vi "HoloLink_get_one_trajectorie.vi"(8 "error in (no error)":errorcluster, 10 "feature_number":i32, 11 "session in":refnum<k35>) -> (0 "error out":errorcluster, 2 "trajectorie":dbl[][](array[numeric]), 3 "Refnum out":refnum<k35>)   [LabVIEW 2023, in "holoPyTracks.lvlib"]
uses:
  holoPyTracks.lvlib
panel:
  # "wavelenght, optical_index, image_size_X, image_size_Y, pixel_size, magnification = holo_info\n\n    propag_param, focus_param, binarisation_param, CCL_param = analyse_parameters\n    distance_ini, nb_plane, propag_step, filter = propag_param\n    high_pass_filter, low_pass_filter = filter\n    #focus parameters unpacking\n    focus_type, sum_size = focus_param\n    #binarisation parameters unpacking\n    nbStdVarThreshold, threshold_target = binarisation_param\n    #CCL parameters unpacking\n    n_connectivity, min_voxel, max_voxel = CCL_param"
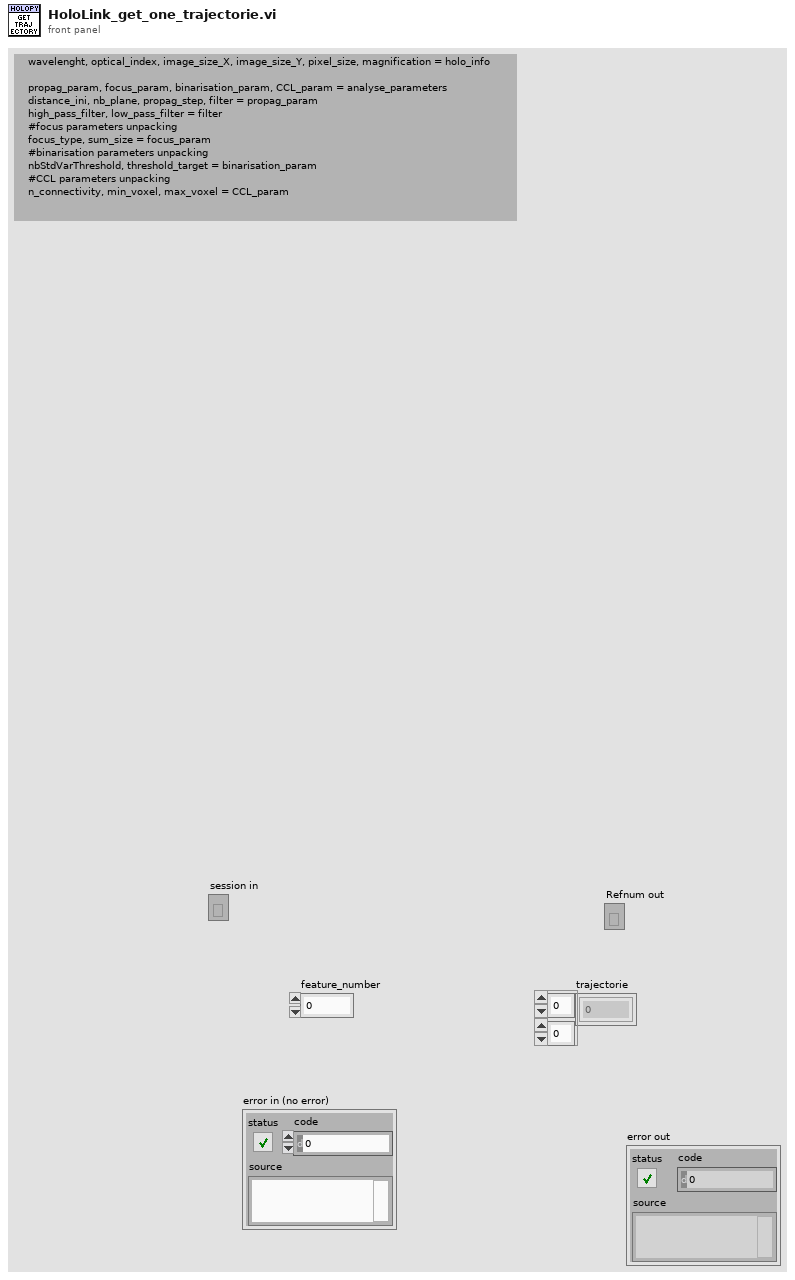
[diagram p1: front panel]
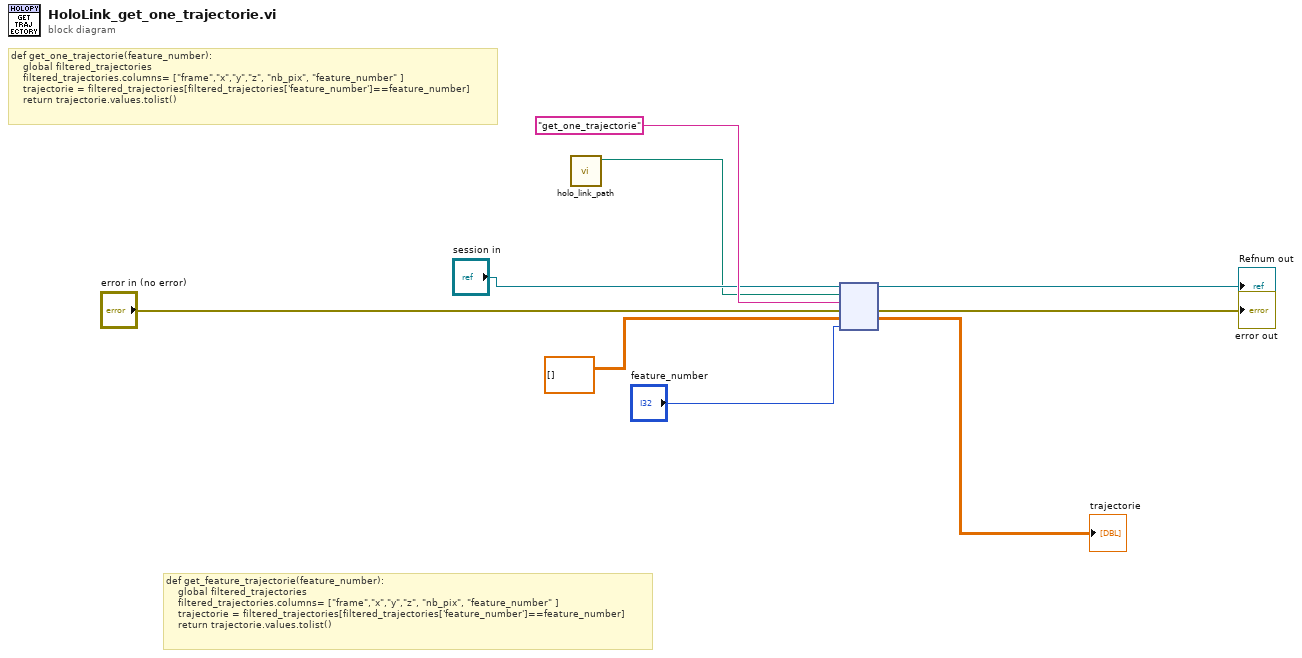
[diagram p0: block diagram]
diagram:
  # "def get_one_trajectorie(feature_number):\n    global filtered_trajectories\n    filtered_trajectories.columns= [\"frame\",\"x\",\"y\",\"z\", \"nb_pix\", \"feature_number\" ]\n    trajectorie = filtered_trajectories[filtered_trajectories['feature_number']==feature_number]\n    return trajectorie.values.tolist()"
  # "def get_feature_trajectorie(feature_number):\n    global filtered_trajectories\n    filtered_trajectories.columns= [\"frame\",\"x\",\"y\",\"z\", \"nb_pix\", \"feature_number\" ]\n    trajectorie = filtered_trajectories[filtered_trajectories['feature_number']==feature_number]\n    return trajectorie.values.tolist()"
  n1 = call "holo_link_path.vi"() -> ("appended path"=w6:path)  [unwired: 11 in]
  n2 = node("session in", w6, "get_one_trajectorie" ("function name"), "error in (no error)", dbl[][] [], "feature_number") -> (→"Refnum out":refnum<k35>, →"error out":errorcluster, →"trajectorie":dbl[][])  [unwired: 1 in, 2 out]
